vi "radius_neighbors.vi"(8 "error in (no error)":errorcluster caption="entrée d'erreur (pas d'erreur)", 11 "RNeighbors.lvclass":refnum<class "RNeighbors.lvclass">) -> (0 "error out":errorcluster caption="sortie d'erreur", 2 "out":T1, 3 "RNeighbors.lvclass 2":refnum<class "RNeighbors.lvclass">)   [LabVIEW 2020, in "RNeighbors.lvclass"]
doc: "Finds the neighbors within a given radius of a point or points.\n\nReturn the indices and distances of each point from the dataset lying in a ball with size radius around the points of the query array. Points lying on the boundary are included in the results.\n\nThe result points are not necessarily sorted by distance to their query point.\n\nParameters\nX : array-like of (n_samples, n_features), default=None\nThe query point or points. If not provided, neighbors of each indexed point are returned. In this case, the query point is not considered its own neighbor.\n\nradius : float, default=None\nLimiting distance of neighbors to return. The default is the value passed to the constructor.\n\nreturn_distance : bool, default=True\nWhether or not to return the distances.\n\nsort_results : bool, default=False\nIf True, the distances and indices will be sorted by increasing distances before being returned. If False, the results may not be sorted. If return_distance=False, setting sort_results=True will result in an error."
uses:
  RNeighbors.lvclass
  C:/Users/cipop/TDF Dropbox/2_Technologies de France/1 - Services et Etudes/PLAIY/2 - DEV/PLAIYLAB/code/Python/Python.lvclass
  C:/Users/cipop/TDF Dropbox/2_Technologies de France/1 - Services et Etudes/PLAIY/2 - DEV/PLAIYLAB/code/Model/Model.lvclass
  C:/Users/cipop/TDF Dropbox/2_Technologies de France/1 - Services et Etudes/PLAIY/2 - DEV/PLAIYLAB/code/Model/Supervised/Neighbors/Neighbors.lvclass
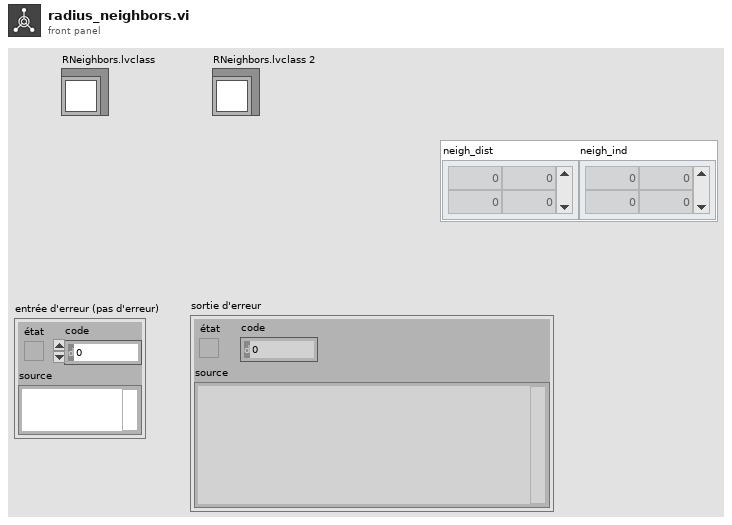
[diagram p1: front panel]
types:
  T1 = cluster{"neigh_dist":dbl[][], "neigh_ind":dbl[][]}
  T2 = typedef "data.ctl" = cluster{"name":string, "X":dbl[][]}
  T3 = typedef "neighbors_data.ctl" = cluster{"y":dbl[][], "sample_weight":dbl[]}
  T4 = typedef "rneighbors_data.ctl" = cluster{"radius":dbl, "mode":string, "return_distance":bool, "sort_results":bool}
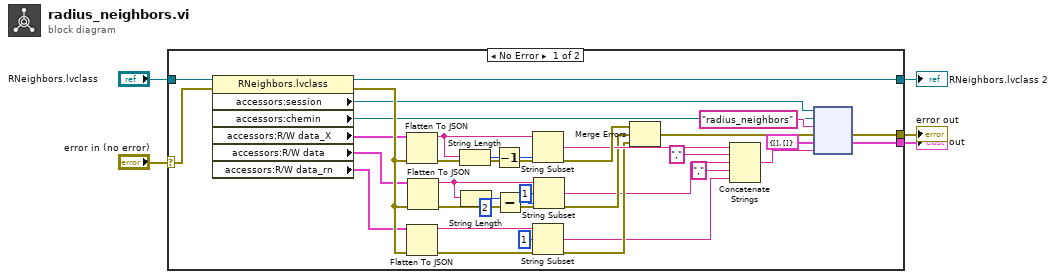
[diagram p0: block diagram]
diagram:
  n1 = case shown="No Error" "error in (no error)" {
    selector: "error in (no error)" -> [w36 w40]
    tunnel: [w37 w40] -> w2
    tunnel: [w6 w39] -> w3
    tunnel: "RNeighbors.lvclass" -> [w35 w39]
    tunnel: [w24 _] -> w1
    frame No Error {
      n2 = property class="RNeighbors.lvclass"(reference=w35, error in=w36) -> (reference out=w6:refnum<class "RNeighbors.lvclass">, error out=w22:errorcluster, "accessors:session"=w9:refnum<k35>, "accessors:chemin"=w8:path, "accessors:R/W data_X"=w11:T2, "accessors:R/W data"=w10:T3, "accessors:R/W data_rn"=w14:T4)
      n3 = Flatten To JSON(anything=w11, error in (no error)=w22) -> (JSON string=w32:string, 11:w29:errorcluster)  [unwired: 1 in]
      n4 = Flatten To JSON(anything=w14, error in (no error)=w22) -> (JSON string=w30:string, 11:w20:errorcluster)  [unwired: 1 in]
      n5 = Flatten To JSON(anything=w10, error in (no error)=w22) -> (JSON string=w18:string, 11:w19:errorcluster)  [unwired: 1 in]
      n6 = String Length(string=w32) -> (length=w34:i32)
      n7 = String Length(string=w18) -> (length=w13:i32)
      n8 = Decrement(x=w34) -> (x-1=w33:i32)
      n9 = Subtract(x=w13, y=2) -> (x-y=w23:i32)
      n10 = String Subset(string=w32, length (rest)=w33) -> (substring=w27:string)  [unwired: 1 in]
      n11 = String Subset(string=w30, offset (0)=1) -> (substring=w15:string)  [unwired: 1 in]
      n12 = String Subset(string=w18, offset (0)=1, length (rest)=w23) -> (substring=w17:string)
      n13 = Merge Errors(w29, w19, w20) -> (w7:errorcluster)
      n14 = Concatenate Strings(w27, "," ("string"), w17, "," ("string"), w15) -> (w26:string)
      n15 = node(w9, w8, "radius_neighbors" ("nom de la fonction"), w7, T1 {"neigh_dist"=[], "neigh_ind"=[]} ("out"), w26) -> (w37:errorcluster, w24:T1)  [unwired: 1 in, 3 out]
    }
    frame Error {
    }
  }
  "error out" <- w2
  "RNeighbors.lvclass 2" <- w3
  "out" <- w1
